vi "Read_PHD_FromJSON_2020-11-06.vi"(5 "MAX Event Rate":dbl=0.05 format="%#_13g", 7 "MIN Event Rate":dbl=0.001 format="%#_13g", 11 "file (use dialog)":path) -> (1 "Average SIS from Filtered Data":cluster{dbl[], dbl[]}(graph), 3 "Filtered SIS Hist in mV-ns":dbl[](array[numeric]))   [LabVIEW 2018]
uses:
  <vilib>/Analysis/NI_AALPro.lvlib
panel:
  out "Original SIS Data":T1
  out "AverageSis":dbl
  out "SpectrumCount":dbl
  out "m/z in SIS Hist":dbl[](array[numeric])
  out "User Filtered SIS Hist":T2(graph)
  out "Nbr Profiles":i32
  out "Profiles":T3(array[cluster])
  out "Original SIS Histogram":cluster{"Intensity":dbl[], "Frequency":dbl[]}(graph)
  out "JSON Text":string
  # "USER Filtering of SIS histogram data"
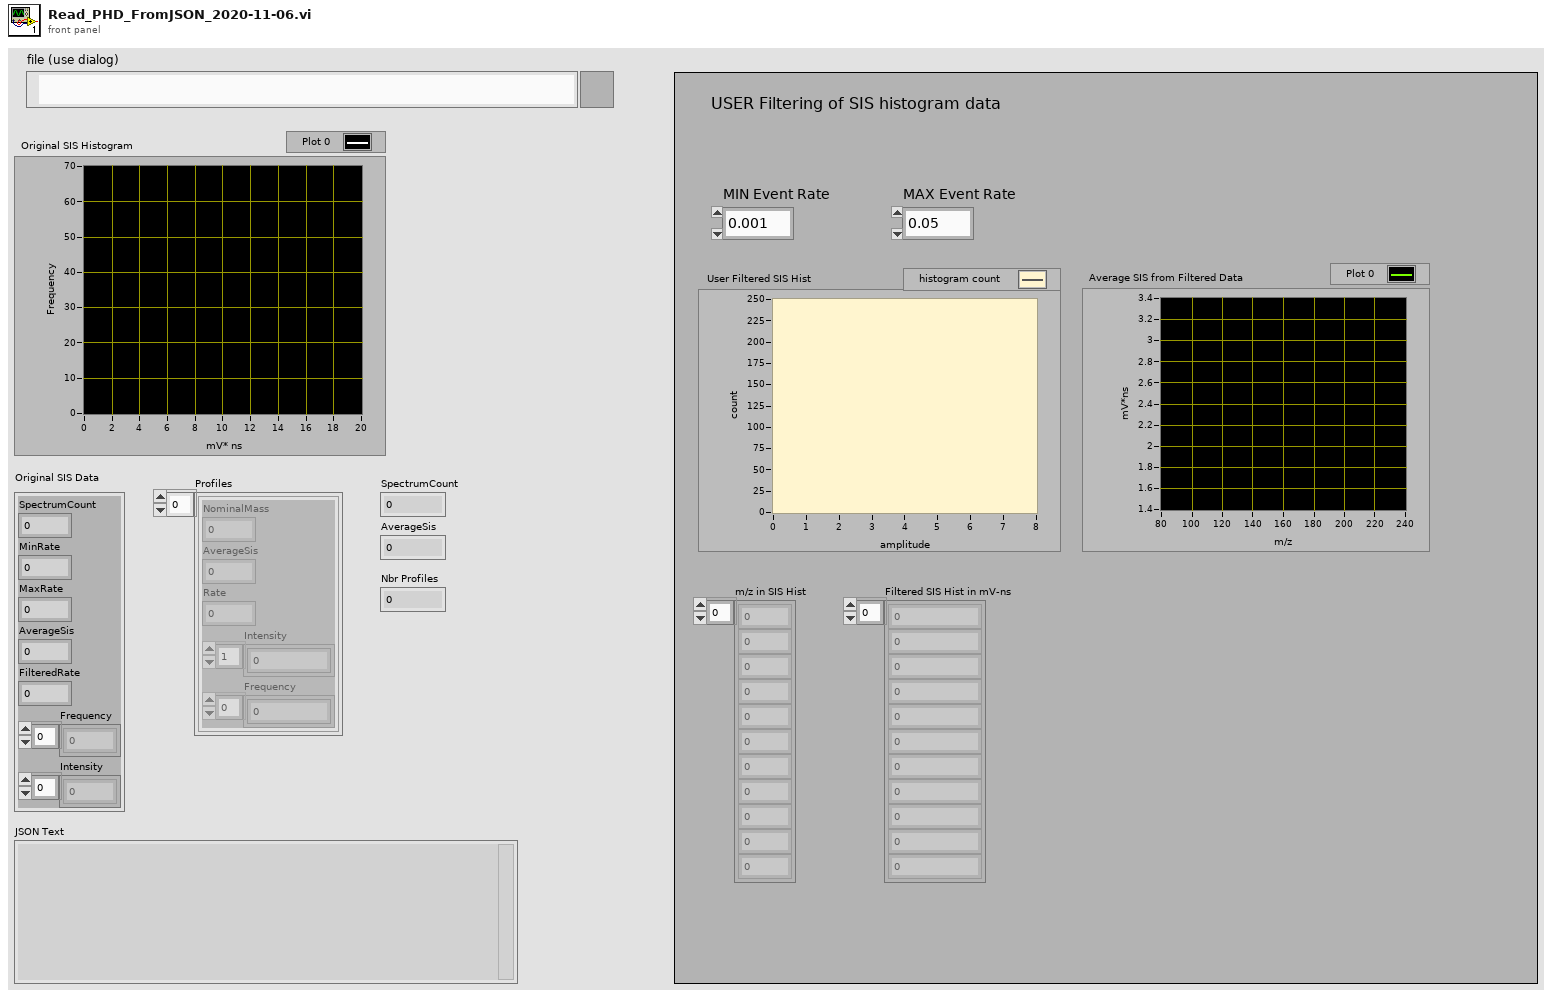
[diagram p1: front panel]
types:
  T1 = cluster{"SpectrumCount":dbl, "MinRate":dbl, "MaxRate":dbl, "AverageSis":dbl, "FilteredRate":dbl, "Frequency":dbl[], "Intensity":dbl[]}
  T2 = cluster{"X Values":dbl[], "Histogram: h(x)":i32[]}
  T3 = cluster{"NominalMass":dbl, "AverageSis":dbl, "Rate":dbl, "Intensity":dbl[], "Frequency":dbl[]}[]
  T4 = cluster{"Profiles":cluster{"NominalMass":dbl, "AverageSis":dbl, "Rate":dbl, "Intensity":dbl[], "Frequency":i32[]}[]}
  T5 = cluster{"NominalMass":dbl, "AverageSis":dbl, "Rate":dbl, "Intensity":dbl[], "Frequency":i32[]}[]
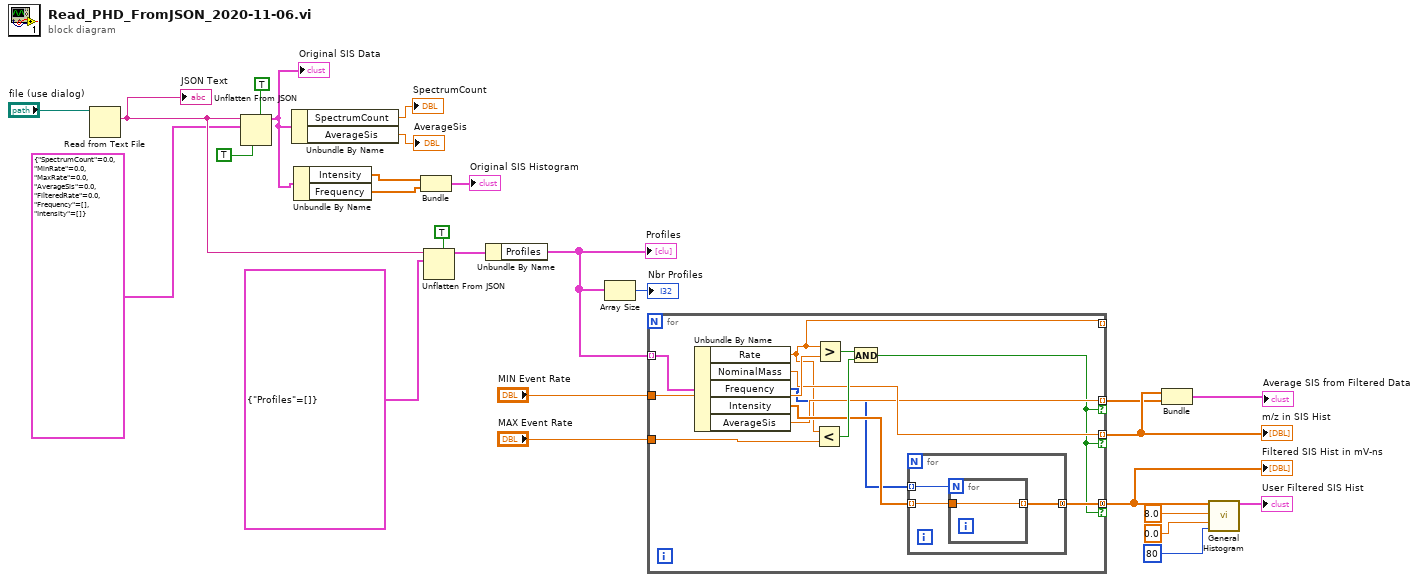
[diagram p0: block diagram]
diagram:
  n1 = Read from Text File(file (use dialog)="file (use dialog)") -> (text=w22:string)  [unwired: 3 in, 3 out]
  "JSON Text" <- w22
  n2 = Unflatten From JSON(enable LabVIEW extensions? (T)=TRUE, JSON string=w22, type and defaults=T1 {"SpectrumCount"=0.0, "MinRate"=0.0, "MaxRate"=0.0, "AverageSis"=0.0, "FilteredRate"=0.0, "Frequency"=[], "Intensity"=[]}, default null elements? (F)=TRUE) -> (value=w2:T1)  [unwired: 3 in, 1 out]
  "Original SIS Data" <- w2
  n3 = Unbundle By Name(w2) -> ("SpectrumCount"=→"SpectrumCount":dbl, "AverageSis"=→"AverageSis":dbl)
  n4 = Unbundle By Name(w2) -> ("Intensity"=w7:dbl[], "Frequency"=w6:dbl[])
  n5 = Bundle("Intensity"=w7, "Frequency"=w6) -> (→"Original SIS Histogram":cluster{"Intensity":dbl[], "Frequency":dbl[]})  [unwired: 1 in]
  n6 = Unflatten From JSON(enable LabVIEW extensions? (T)=TRUE, JSON string=w22, type and defaults=T4 {"Profiles"=[]}) -> (value=w19:T4)  [unwired: 4 in, 1 out]
  n7 = Unbundle By Name(w19) -> ("Profiles"=w18:T5)
  "Profiles" <- w18
  n8 = Array Size(array=w18) -> (size(s)=→"Nbr Profiles":i32)
  n9 = for {
    tunnel: w18 -> [w38] mode=indexing
    tunnel: "MIN Event Rate" -> [w36]
    tunnel: "MAX Event Rate" -> [w35]
    tunnel: [w33] -> w10 mode=indexing if=w29
    tunnel: [w31] -> w15 mode=concatenating if=w29
    tunnel: [w30] -> w9 mode=indexing if=w29
    tunnel: [w28] -> _ mode=indexing
    n10 = Unbundle By Name(w38) -> ("Rate"=w28:dbl, "NominalMass"=w33:dbl, "Frequency"=w27:i32[], "Intensity"=w32:dbl[], "AverageSis"=w30:dbl)
    n11 = Less?(x=w28, y=w35) -> (x < y?=w34:bool)
    n12 = Greater?(x=w28, y=w36) -> (0:w37:bool)
    n13 = And(x=w37, y=w34) -> (x .and. y?=w29:bool)
    n14 = for {
      tunnel: w27 -> [w39] mode=indexing
      tunnel: w32 -> [w41] mode=indexing
      tunnel: [w40] -> w31 mode=concatenating
      n15 = for {
        N: w39 -> [_]
        tunnel: w41 -> [w42]
        tunnel: [w42] -> w40 mode=indexing
      }
    }
  }
  "m/z in SIS Hist" <- w10
  "Filtered SIS Hist in mV-ns" <- w15
  n16 = Bundle(w10, w9) -> (→"Average SIS from Filtered Data":cluster{dbl[], dbl[]})  [unwired: 1 in]
  n17 = call <vilib>:"General Histogram.vi"("X"=w15, "max"=8.0, "min"=0.0, "# bins"=80) -> ("Histogram Graph"=→"User Filtered SIS Hist":T2)  [unwired: 7 in, 4 out]
